vi "TIFF_1_OpenSourceImage.vi"(8 "error in (no error)":errorcluster, 11 "Source File Image Path":path=path "C:/Users/Sebastien/Documents/GitHub/LABVIEW-Useful-codes/TIFF/Test_Image_1.tif") -> (0 "Error Out":errorcluster, 3 "output cluster":T1)   [LabVIEW 2025]
doc: "This software was created to prototype writing metadata to a TIFF file with a single image.\n\n<B>Usage:</B> This software is free to use, copy or plagiariaze. It is provided \"as-is\", and no technical support will be provided. The copyright is retained by NASA Marshall Space Flight Center.\n\n<B>Testing:</B> This software was tested by A) verifying that operations were completed successfully using LabVIEW 2009 on Windows XP, .NET version 4.0 and B) Windows Vista Microsoft Office Picture Manager was able to read and display the output file and C) Windows Vista Windows Photo Gallery was able to read and display the output file and the Description and D) Adobe Photoshop for Macintosh was able to correctly load and display the image and all the metadata.\n\n<B>Note:</B> This software requires .NET version 4.0\n\n<B>Warning:</B> This software will overwrite the destination file if it exists.\n\nThis software originally developed by:\nDerek Mayer\nBAE Systems - Technology Solutions & Services\n308 Voyager Way\nHuntsville, AL 35806\n(256) 890-8000\nwww.mevatec.com\nwww.baesystems.com/TSS\nSeptember 2010"
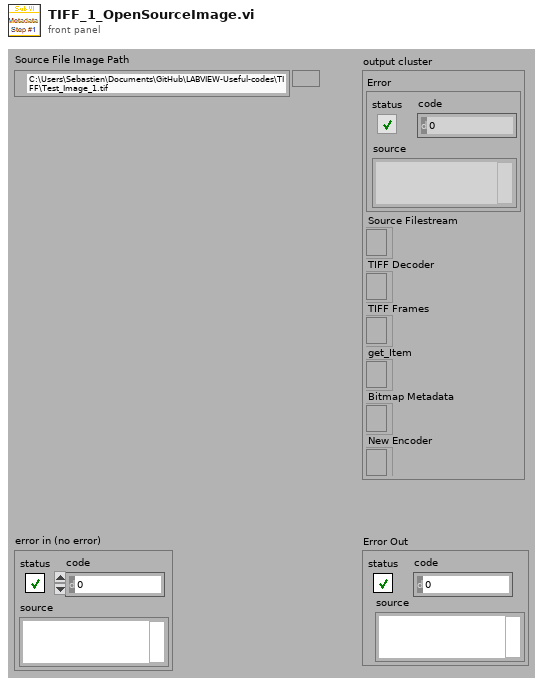
[diagram p1: front panel]
types:
  T1 = cluster{"Error":errorcluster, "Source Filestream":refnum<k24>, "TIFF Decoder":refnum<k24>, "TIFF Frames":refnum<k24>, "get_Item":refnum<k24>, "Bitmap Metadata":refnum<k24>, "New Encoder":refnum<k24>}
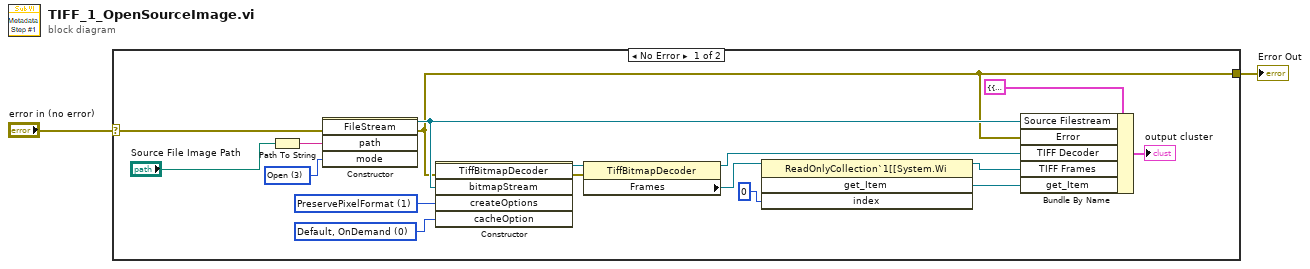
[diagram p0: block diagram]
diagram:
  n1 = case shown="No Error" "error in (no error)" {
    selector: "error in (no error)" -> [w3 w20]
    tunnel: [w4 w20] -> w1
    frame No Error {
      w7 = 0 items=["Default, OnDemand", "OnLoad", "None"] ("cacheOption")
      w8 = 1 items=["None"=0, "PreservePixelFormat"=1, "DelayCreation"=2, "IgnoreColorProfile"=4, "IgnoreImageCache"=8] ("createOptions")
      w5 = 3 items=["CreateNew"=1, "Create"=2, "Open"=3, "OpenOrCreate"=4, "Truncate"=5, "Append"=6] ("mode")
      n2 = Path To String(path="Source File Image Path") -> (string=w11:string)
      n3 = constructor class="FileStream"(error in=w3, "path"=w11, "mode"=w5) -> (reference out=w15:refnum<k24>, error out=w4:errorcluster)  [unwired: 2 in, 3 out]
      n4 = constructor class="TiffBitmapDecoder"(error in=w4, "bitmapStream"=w15, "createOptions"=w8, "cacheOption"=w7) -> (reference out=w13:refnum<k24>, error out=w12:errorcluster)  [unwired: 2 in, 4 out]
      n5 = property class="TiffBitmapDecoder"(reference=w13, error in=w12) -> (reference out=w16:refnum<k24>, "Frames"=w14:refnum<k24>)  [unwired: 1 out]
      n6 = invoke class="ReadOnlyCollection`1[[System.Wi" method="get_Item"(reference=w14, "index"=0) -> (reference out=w17:refnum<k24>, "get_Item"=w18:refnum<k24>)  [unwired: 2 in, 2 out]
      n7 = Bundle By Name(cluster=T1 {"Error"={"status"=FALSE, "code"=0, "source"=""}, "Source Filestream"=refnum, "TIFF Decoder"=refnum, "TIFF Frames"=refnum, "get_Item"=refnum, "Bitmap Metadata"=refnum, "New Encoder"=refnum}, "Source Filestream"=w15, "Error"=w4, "TIFF Decoder"=w16, "TIFF Frames"=w17, "get_Item"=w18) -> (→"output cluster":T1)
    }
    frame Error {
    }
  }
  "Error Out" <- w1
